vi "Time Stamp to ISO 8601 with milliseconds.vi"(8 "error in (no error)":errorcluster, 11 "Timestamp":timestamp) -> (0 "error out":errorcluster, 3 "ISO 8601 w/ms":string)   [LabVIEW 2013]
doc: "Statnett PMU Reference Library Template VI with open block diagram\nUse this when creating new VIs in your application"
panel:
  # "INPUT"
  # "INTERMEDIATE"
  # "OUTPUT"
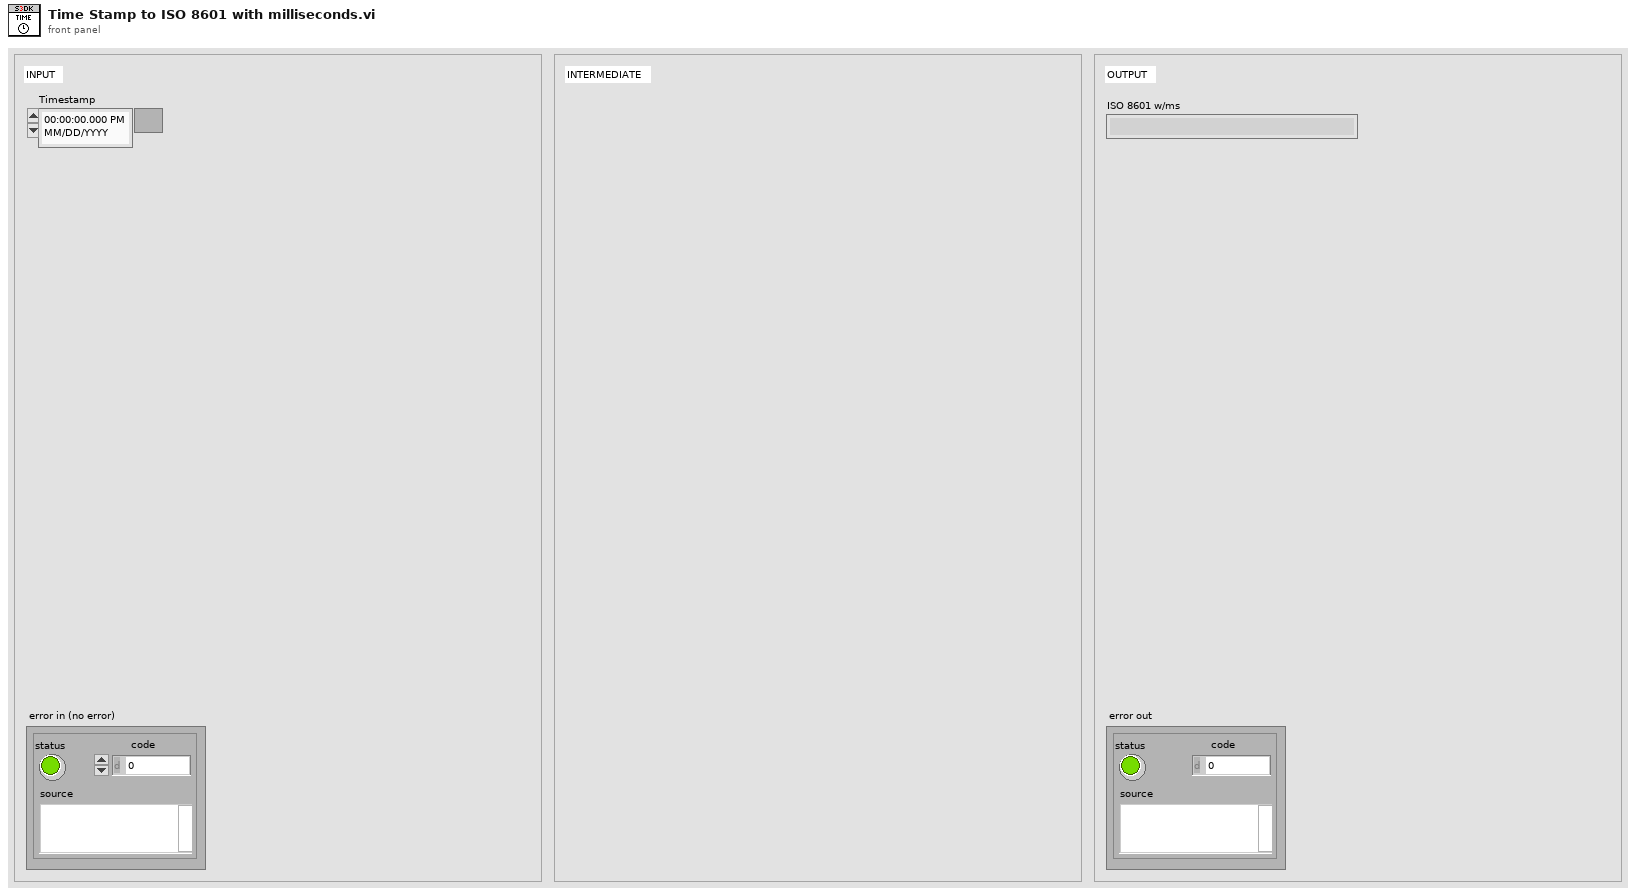
[diagram p1: front panel]
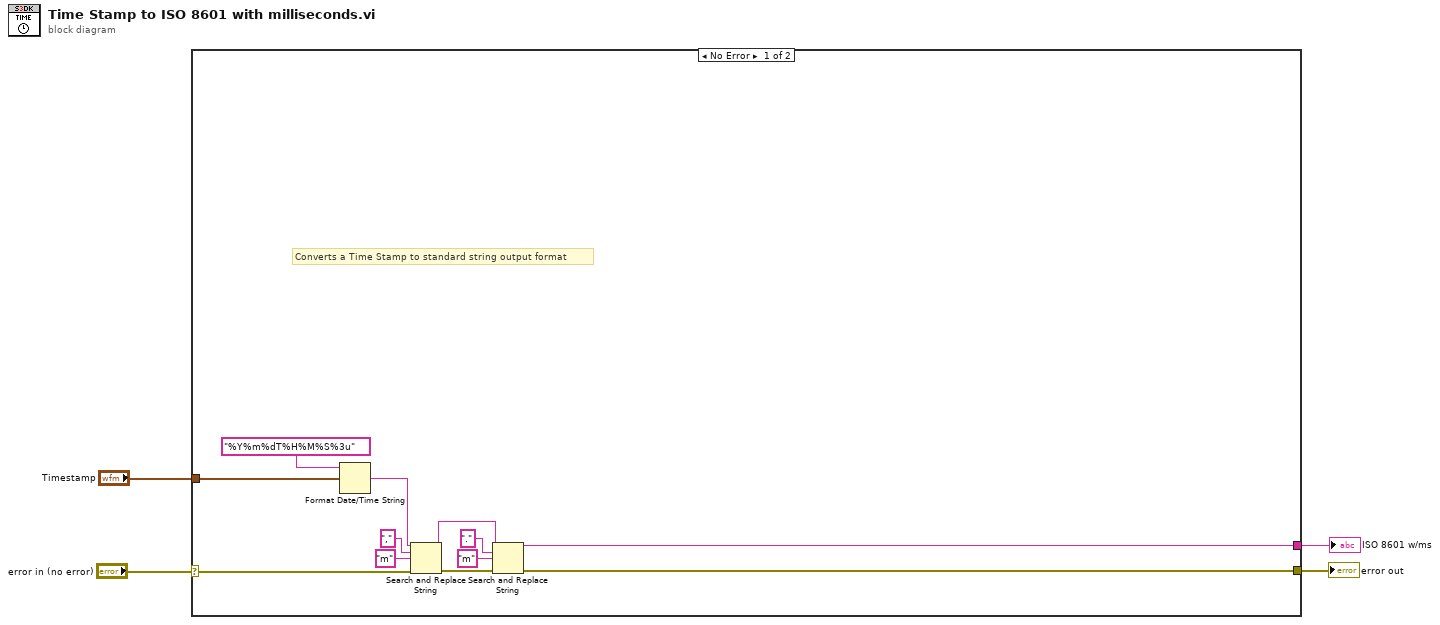
[diagram p0: block diagram]
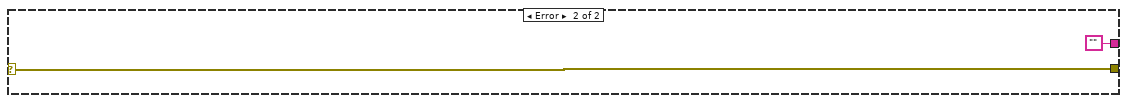
[diagram p2: hidden frame]
diagram:
  n1 = case shown="No Error" "error in (no error)" {
    selector: "error in (no error)" -> [w7 w18]
    tunnel: [w5 w18] -> w3
    tunnel: "Timestamp" -> [w9 _]
    tunnel: [w8 "" ("result string")] -> w1
    frame No Error {
      # "Converts a Time Stamp to standard string output format"
      n2 = Format Date/Time String(time format string (%c)="%Y%m%dT%H%M%S%3u", seconds (now)=w9) -> (date/time string=w15:string)  [unwired: 1 out]
      n3 = Search and Replace String(input string=w15, search string=",", replace string="m" ("replace string (\"\")"), error in=w7) -> (result string=w10:string, error out=w6:errorcluster)  [unwired: 6 out]
      n4 = Search and Replace String(input string=w10, search string=".", replace string="m" ("replace string (\"\")"), error in=w6) -> (result string=w8:string, error out=w5:errorcluster)  [unwired: 6 out]
    }
    frame Error {
    }
  }
  "error out" <- w3
  "ISO 8601 w/ms" <- w1
